vi "Write Control Caption.vi"(8 "error in":errorcluster, 10 "Text":refnum<class "UTF-8 String.lvclass">, 11 "Control Ref":refnum<vi>) -> (0 "error out":errorcluster)   [LabVIEW 2020, in "G-Unicode.lvlib"]
doc: "Write text to a control's caption and display it as unicode. <b>Text</b> can be a UTF-8 String or LabVIEW String."
uses:
  G-Unicode.lvlib
  Types/UTF-8 String/UTF-8 String.lvclass
  Types/UTF-8 String/UTF-8 String.lvclass/UTF-8 String.ctl
  13c16a8b-00d3-486b-99f0-c83eae9facb1.vi
  Private/Conversion/String as Encoded String.vi
  Private/Conversion/Polymorphic VIs/String as Encoded String (UTF-8 String).vi
  Types/UTF-8 String/Read Encoded UTF-8 String.vi
  Private/Conversion/Encoded UTF-8 String to Encoded UTF-16LE String.vi
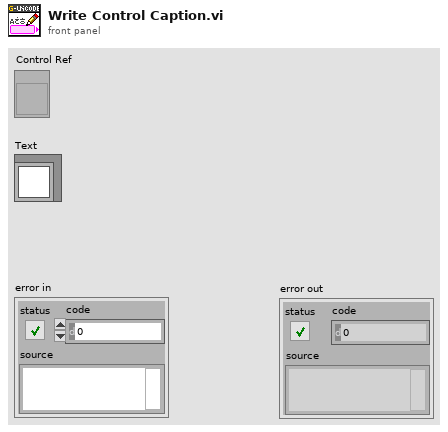
[diagram p1: front panel]
types:
  T1 = typedef "G-Unicode.lvlib/Encoded UTF-16LE String.ctl" = string
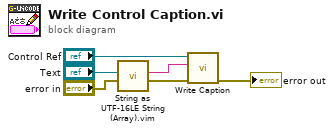
[diagram p0: block diagram]
diagram:
  n1 = call "String as UTF-16LE String (Array).vim"("error in"="error in", "String"="Text") -> ("error out"=w1:errorcluster, "UTF-16LE String"=w3:T1)  [unwired: 8 in]
  n2 = call "Write Caption.vi"("error in"=w1, "Value"=w3, "Control Reference in"="Control Ref") -> ("error out"=→"error out":errorcluster)  [unwired: 7 in, 1 out]
